vi "PPL_SIM_SIM_ODOM_EXECUTE.vi"(8 "error in (no error)":errorcluster) -> (0 "error out":errorcluster)   [LabVIEW 2019]
uses:
  <vilib>/Rock Robotics/WPI/ThirdParty/JAS_Junk/TrajLib/Rotation2d_Minus.vi
  <vilib>/Rock Robotics/WPI/ThirdParty/JAS_Junk/TrajLib/Rotation2d_Plus.vi
  <vilib>/Rock Robotics/WPI/ThirdParty/JAS_Junk/TrajLib/Twist2d_Create.vi
  <vilib>/Rock Robotics/WPI/ThirdParty/JAS_Junk/TrajLib/Rotation2d_GetRadians.vi
  <vilib>/Rock Robotics/WPI/ThirdParty/JAS_Junk/TrajLib/Rotation2d_UnaryMinus.vi
  <vilib>/Rock Robotics/WPI/ThirdParty/JAS_Junk/TrajLib/Rotation2d_RotateBy.vi
  <vilib>/Rock Robotics/WPI/ThirdParty/JAS_Junk/TrajLib/Rotation2d_CreateXY.vi
  <vilib>/Rock Robotics/WPI/ThirdParty/JAS_Junk/TrajLib/Util_CalcDist.vi
  Diff_Drive_System/PPL_DRIVE_GLOBALS.vi
  PPL_SIM_SIM_Globals.vi
  <vilib>/Rock Robotics/WPI/ThirdParty/JAS_Junk/TrajLib/Pose2d_Exp.vi
  <vilib>/Rock Robotics/WPI/ThirdParty/JAS_Junk/TrajLib/Trajectory_Library.lvlib
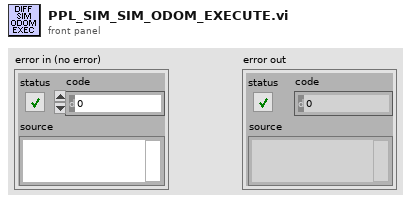
[diagram p1: front panel]
types:
  T1 = typedef "Trajectory_Library.lvlib/DIFF_DRIVE_ODOM2.ctl" = cluster{"M_POSE_Meters":T2, "M_GyroOffset":T4, "M_PrevAngle":T4, "M_PrevLeftDist_M":dbl, "M_PrevRightDist_M":dbl, "M_InitLeftDist_M":dbl, "M_InitRightDist_M":dbl}
  T2 = typedef "Trajectory_Library.lvlib/POSE2D.ctl" = cluster{"TRANSLATION":T3, "ROTATION":T4}
  T3 = typedef "Trajectory_Library.lvlib/TRANSLATION2D.ctl" = cluster{"X":dbl, "Y":dbl}
  T4 = typedef "Trajectory_Library.lvlib/ROTATION2D.ctl" = cluster{"VALUE":dbl, "COS":dbl, "SIN":dbl}
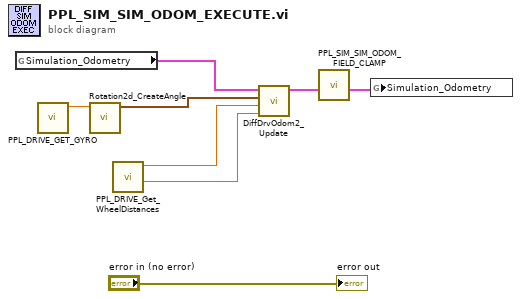
[diagram p0: block diagram]
diagram:
  n1 = global read "PPL_SIM_SIM_Globals.vi" "Simulation_Odometry"() -> (w3:T1)
  n2 = call "PPL_DRIVE_GET_GYRO.vi"() -> ("Gyro Heading Radians"=w5:dbl)  [unwired: 11 in]
  n3 = call <vilib>:"Rotation2d_CreateAngle.vi"("Angle"=w5) -> ("ROTATION"=w8:T4)  [unwired: 10 in]
  n4 = call "PPL_DRIVE_Get_WheelDistances.vi"() -> ("Right Wheel Dist M"=w1:dbl, "Left Wheel Dist M"=w2:dbl)  [unwired: 10 in]
  n5 = call <vilib>:"DiffDrvOdom2_Update.vi"("Right Distance M"=w1, "Left Distance M"=w2, "Gyro Reading"=w8, "In DIFF_DRIVE_ODOM"=w3) -> ("Out DIFF_DRIVE_ODOM"=w7:T1)  [unwired: 6 in, 1 out]
  n6 = call "PPL_SIM_SIM_ODOM_FIELD_CLAMP.vi"("in SWERVE_DRIVE_ODOMETRY"=w7) -> ("out SWERVE_DRIVE_ODOMETRY"=w4:T1)  [unwired: 10 in]
  n7 = global write "PPL_SIM_SIM_Globals.vi" "Simulation_Odometry"(w4) -> ()
  "error out" <- "error in (no error)"
